vi "RateLimiter.vi"(10 "Max dx/dt":dbl=1.0, 11 "Input":dbl(slide) scale=-10.0..10.0) -> (3 "Output":dbl)   [LabVIEW 2016]
doc: "Limits how fast the input changes"
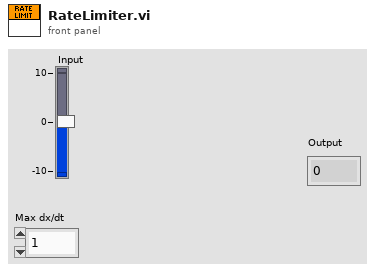
[diagram p1: front panel]
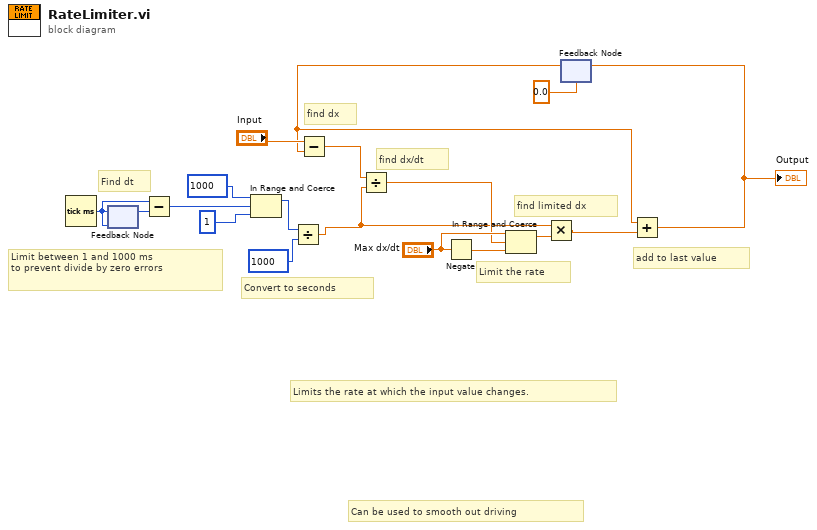
[diagram p0: block diagram]
diagram:
  # "Can be used to smooth out driving"
  # "Limits the rate at which the input value changes."
  # "Convert to seconds"
  # "find limited dx"
  # "add to last value"
  # "Limit the rate"
  # "find dx/dt"
  # "find dx"
  # "Limit between 1 and 1000 ms\nto prevent divide by zero errors"
  # "Find dt"
  n1 = Tick Count (ms)() -> (millisecond timer value=w17:u32)
  n2 = feedback-in #1(w17) -> ()
  n3 = feedback #1(w17) -> (w18:u32)
  n4 = Subtract(x=w17, y=w18) -> (x-y=w4:u32)
  n5 = In Range and Coerce(upper limit=u32 1000, x=w4, lower limit=u32 1) -> (coerced(x)=w1:u32)  [unwired: 1 out]
  n6 = Divide(x=w1, y=u32 1000) -> (x/y=w5:dbl)
  n7 = Negate(x="Max dx/dt") -> (-x=w15:dbl)
  n8 = feedback #2(0.0 ("x-y")) -> (w11:dbl)
  n9 = Subtract(x="Input", y=w11) -> (x-y=w10:dbl)
  n10 = Divide(x=w10, y=w5) -> (x/y=w9:dbl)
  n11 = In Range and Coerce(upper limit="Max dx/dt", x=w9, lower limit=w15) -> (coerced(x)=w7:dbl)  [unwired: 1 out]
  n12 = Multiply(x=w5, y=w7) -> (x*y=w6:dbl)
  n13 = Add(x=w11, y=w6) -> (x+y=w8:dbl)
  "Output" <- w8
  n14 = feedback-in #2(w8) -> ()
